vi "check errors exist or not.vi"(8 "error in":errorcluster, 11 "judge column":string[](array[string])) -> (0 "error out":errorcluster, 3 "Go on?":bool)   [LabVIEW 2010]
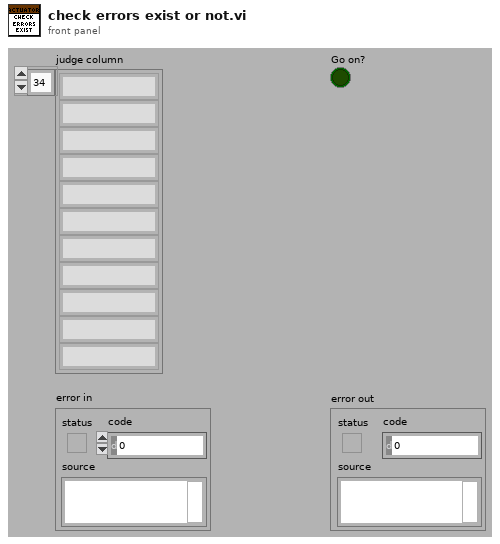
[diagram p1: front panel]
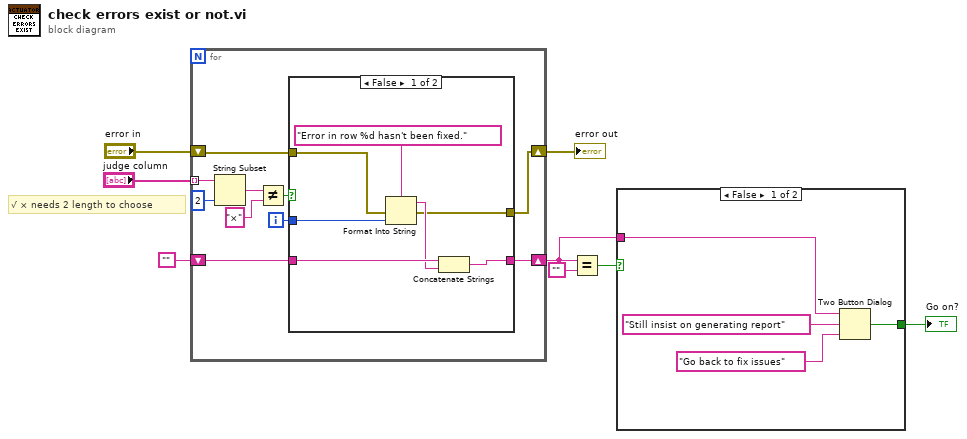
[diagram p0: block diagram]
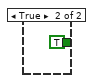
[diagram p2: hidden frame]
diagram:
  # "√ × needs 2 length to choose"
  n1 = for {
    tunnel: "judge column" -> [w18] mode=indexing
    shift-right: [w13] -> w2
    shift-left: "" -> [w14]
    shift-right: [w10] -> w5
    shift-left: "error in" -> [w11]
    i -> [w12]
    n2 = String Subset(string=w18, length (rest)=2 ("length (rest)")) -> (substring=w9:string)  [unwired: 1 in]
    n3 = Not Equal?(x=w9, y="×") -> (x != y?=w15:bool)
    n4 = case shown="False" w15 {
      tunnel: w14 -> [w23 w27]
      tunnel: [w21 w27] -> w13
      tunnel: w12 -> [w24 _]
      tunnel: w11 -> [w20 w26]
      tunnel: [w19 w26] -> w10
      frame False {
        n5 = Format Into String(format string="Error in row %d hasn't been fixed.", error in=w20, w24) -> (resulting string=w22:string, error out=w19:errorcluster)  [unwired: 1 in]
        n6 = Concatenate Strings(w23, w22) -> (w21:string)
      }
      frame True {
      }
    }
  }
  "error out" <- w5
  n7 = Equal?(x=w2, y="") -> (x = y?=w3:bool)
  n8 = case shown="False" w3 {
    tunnel: w2 -> [w29 _]
    tunnel: [w28 TRUE ("T button?")] -> w1
    frame False {
      n9 = Two Button Dialog(message=w29, 1:"Go back to fix issues" ("F button name (\"Cancel\")"), 2:"Still insist on generating report" ("T button name (\"OK\")")) -> (T button?=w28:bool)
    }
    frame True {
    }
  }
  "Go on?" <- w1
